vi "GUI_BELLA_PlL2PresCtl.vi"() -> ()   [LabVIEW 2013]
uses:
  Shared/GUI_Template/GUI_master/tcp_new_data_event.ctl
  Shared/GUI_Template/GUI_master/tcp new data cluster.ctl
panel:
  out "tcp data event":T1
  in  "Refresh Button":bool
  in  "Select device":string(combo)="PL1-PresCtl"
  in  "PressureSetPoint.device 2::1":dbl=0.001 caption="Pressure Set Point Plasma1 LP" min=0.0 max=20.0 format="%_4f"
  in  "PressureReading.device 2::1":dbl=0.001 caption="Pressure Reading Plasma1 LP" min=-10.0 max=20.0 format="%_4p"
  in  "stop":bool
  in  "PressureSetPoint.device 1::1":dbl=0.001 caption="Pressure Set Point Plasma1 HP" min=0.0 max=20.0 format="%_4f"
  in  "PressureReading.device 1::1":dbl=0.001 caption="Pressure Reading Plasma1 HP" min=-10.0 max=20.0 format="%_4p"
  in  "GUIdevice 1":string="PL2-PresCtl"
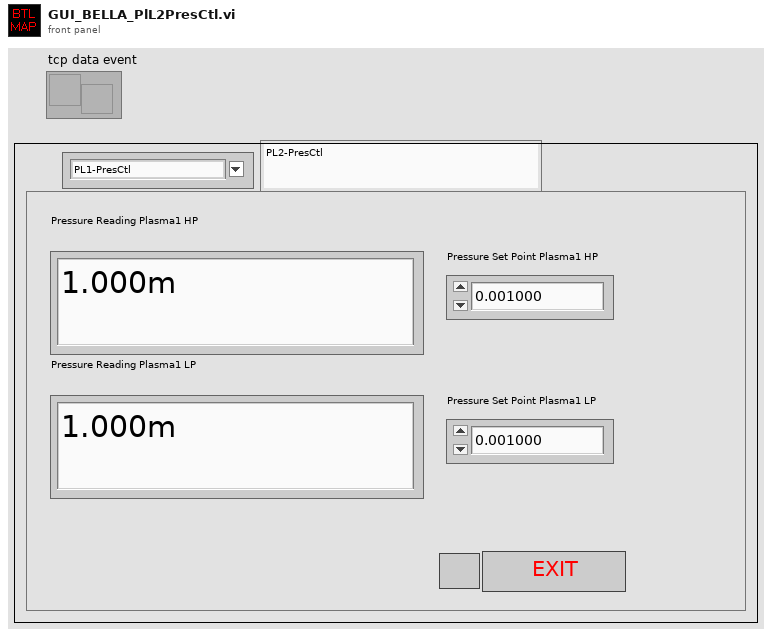
[diagram p1: front panel]
types:
  T1 = typedef "tcp_new_data_event.ctl" = refnum<user-event>
  T2 = enum32{"invalid app kind", "Development System", "Run Time System", "Student Edition", "Embedded LabVIEW", "Evaluation", "Custom"}
  T3 = typedef "tcp new data cluster.ctl" = cluster{"EventEnum":enum16{"new data", "connection status update"}, "Device name":string}
  T4 = enum32{"Invalid", "Standard", "Closed", "Hidden", "Minimized", "Maximized"}
  T5 = cluster{"Core":cluster{"Current VI Reference":refnum<vi>, "Close Panel on Exit?":bool}, "Your Boolean data":bool, "Your string data":string, "SuperGUI":cluster{"STOP queue":refnum<queue>, "SuperGUI ref":refnum<vi>}}
  T6 = cluster{"STOP queue":refnum<queue>, "SuperGUI ref":refnum<vi>}
  T7 = cluster{"Current VI Reference":refnum<vi>, "Close Panel on Exit?":bool}
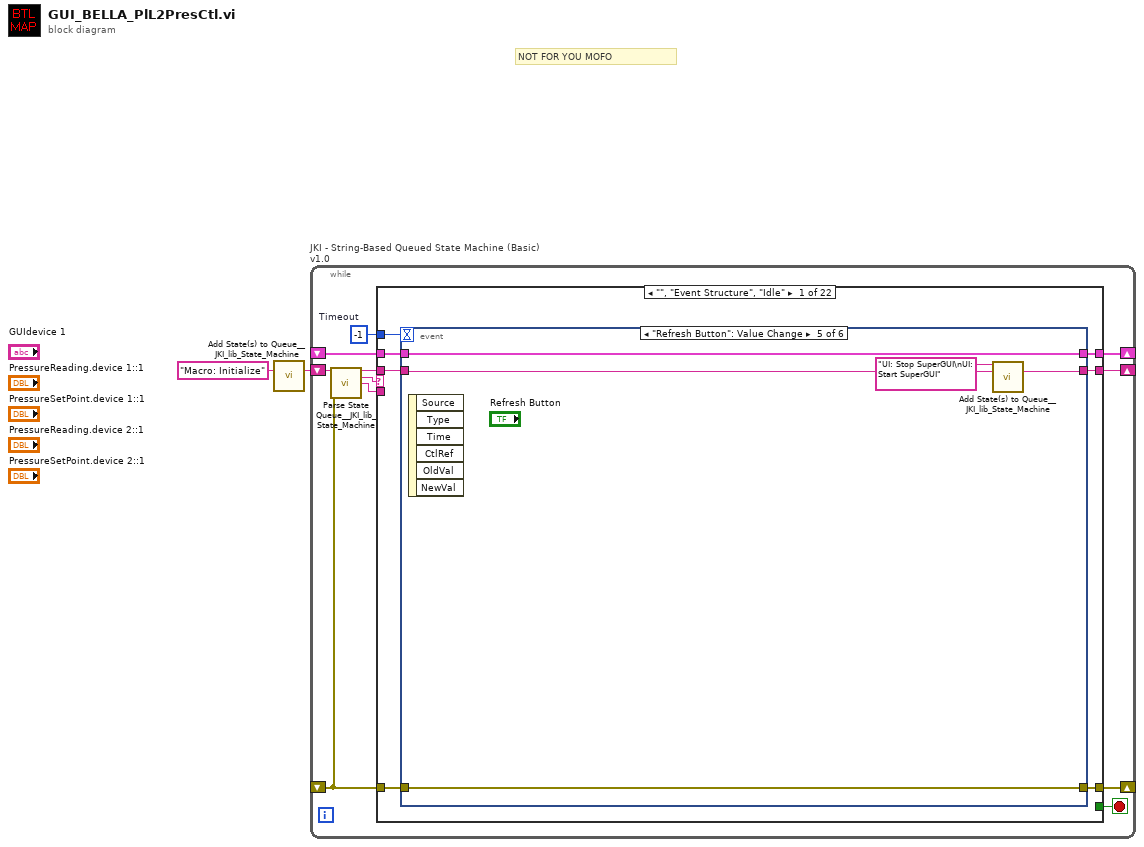
[diagram p0: block diagram]
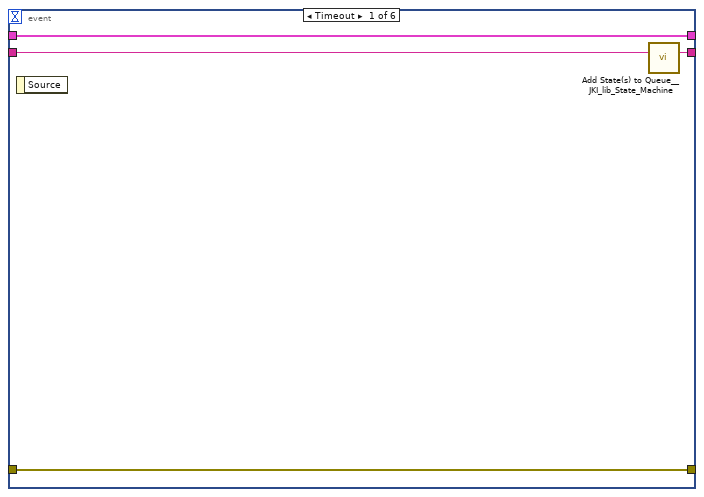
[diagram p2: hidden frame]
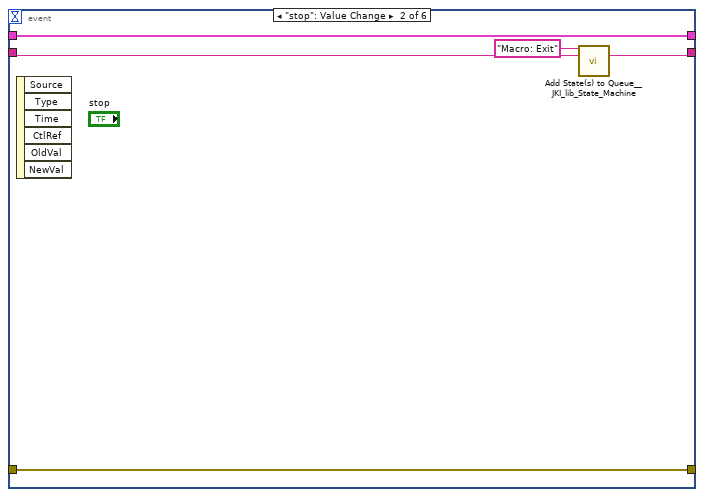
[diagram p3: hidden frame]
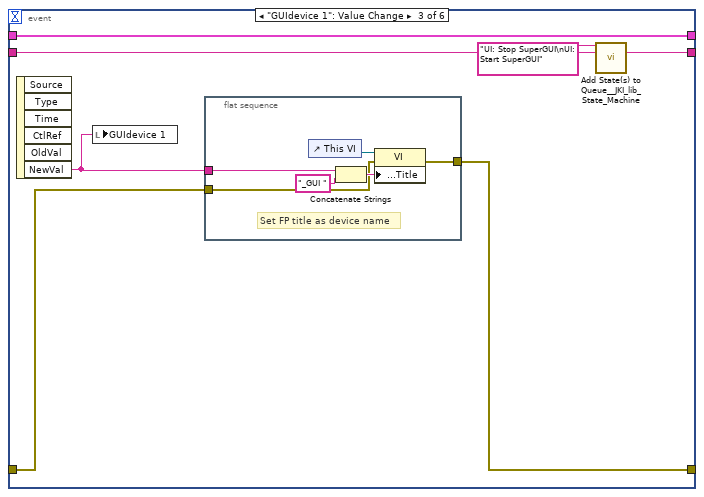
[diagram p4: hidden frame]
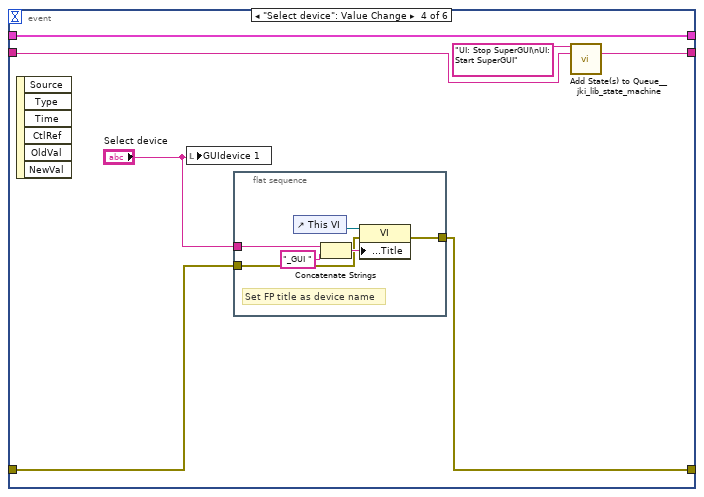
[diagram p5: hidden frame]
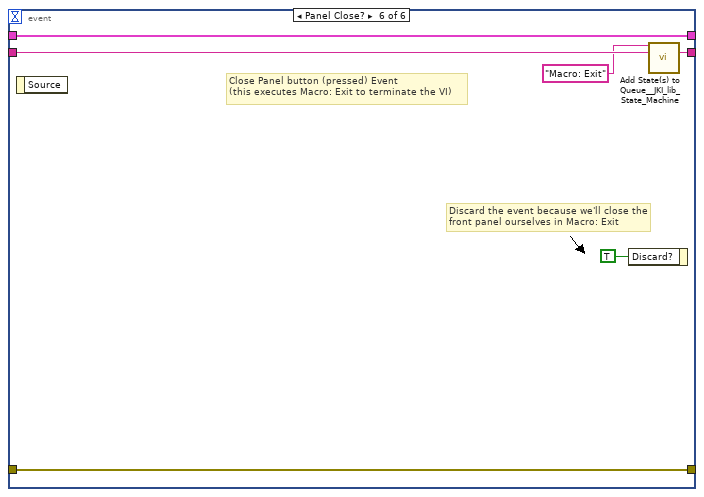
[diagram p6: hidden frame]
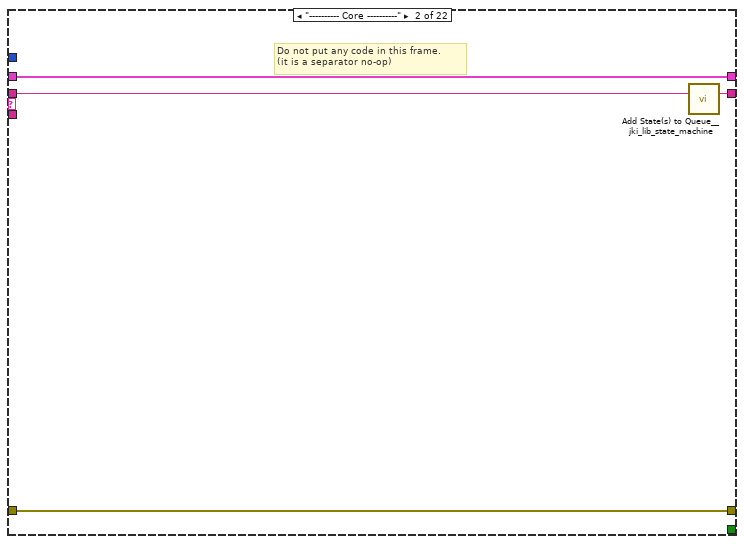
[diagram p7: hidden frame]
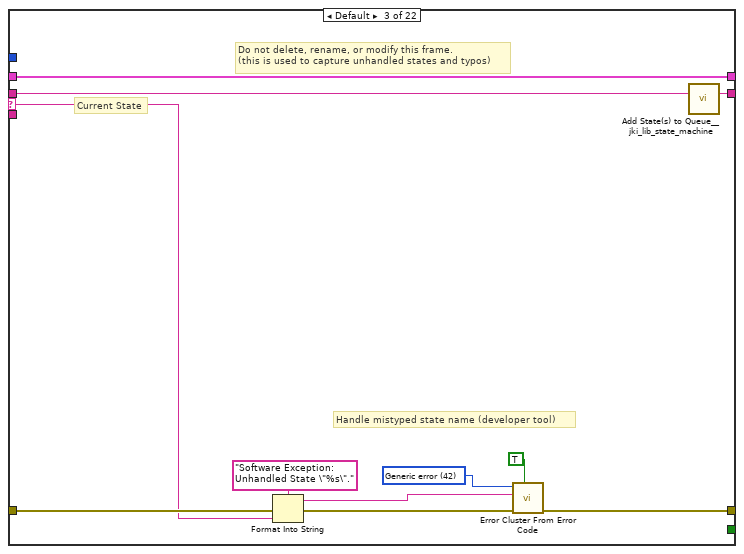
[diagram p8: hidden frame]
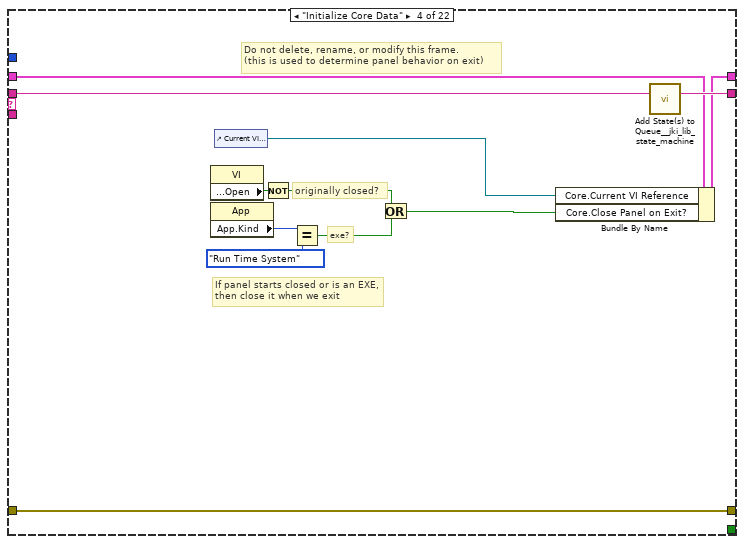
[diagram p9: hidden frame]
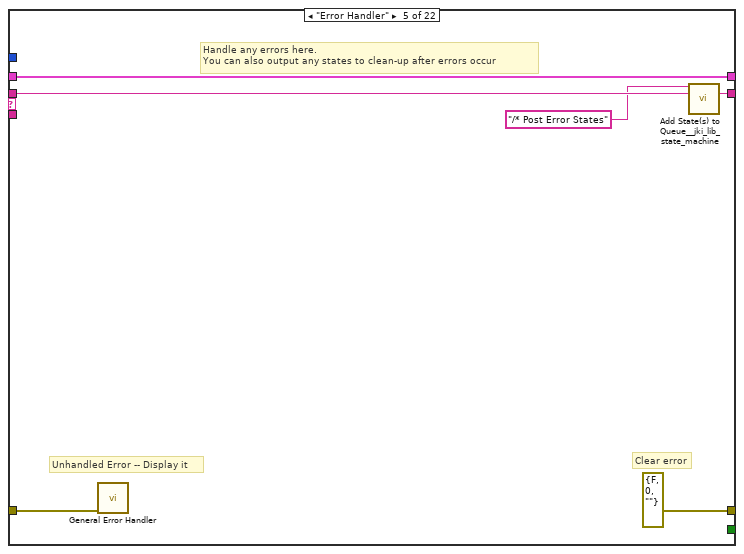
[diagram p10: hidden frame]
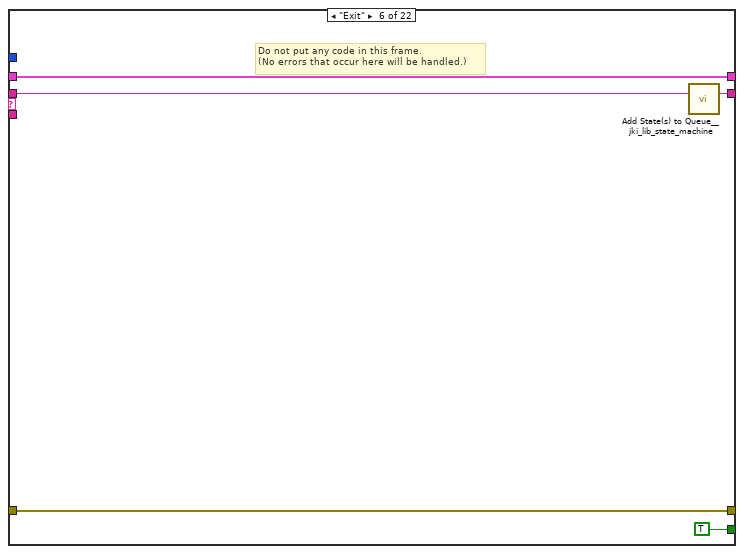
[diagram p11: hidden frame]
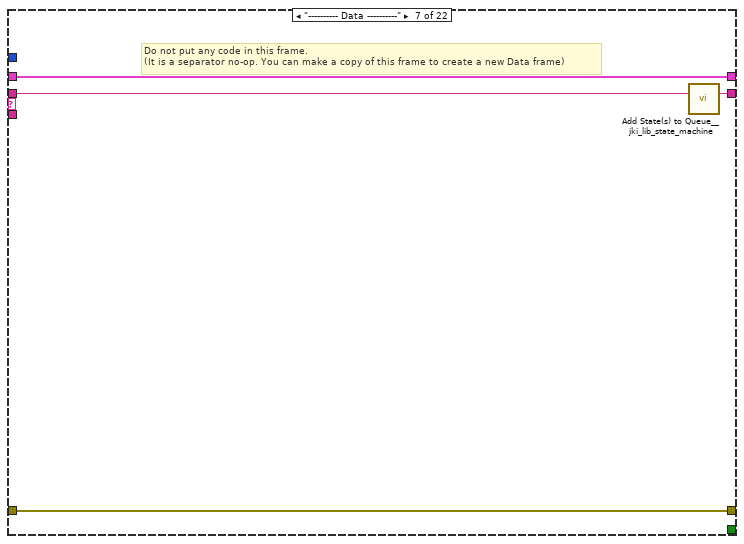
[diagram p12: hidden frame]
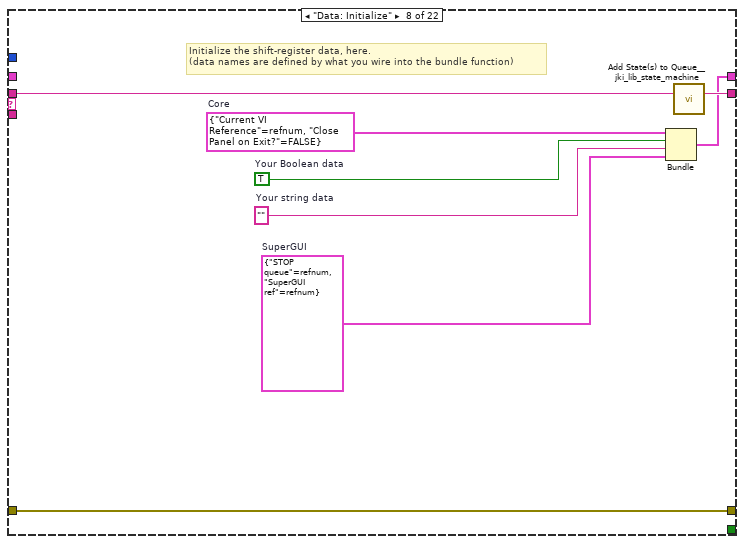
[diagram p13: hidden frame]
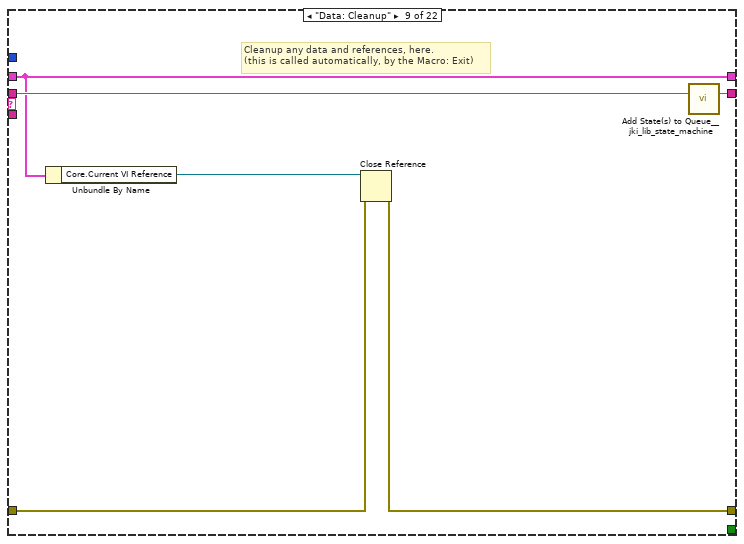
[diagram p14: hidden frame]
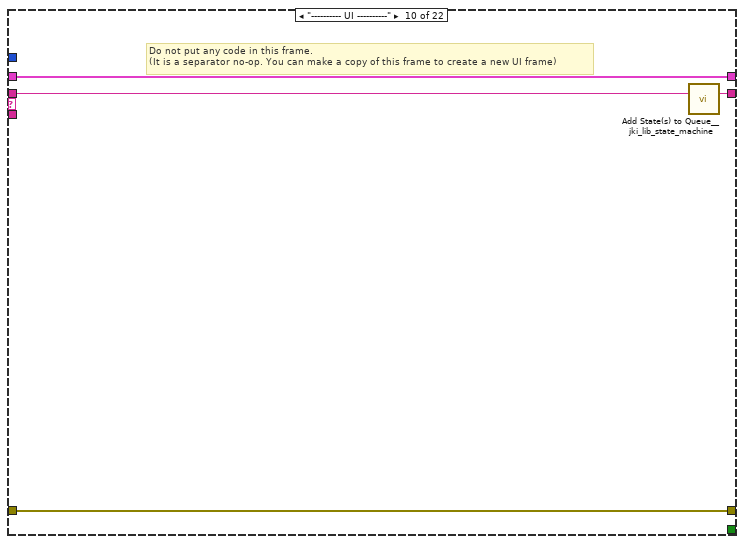
[diagram p15: hidden frame]
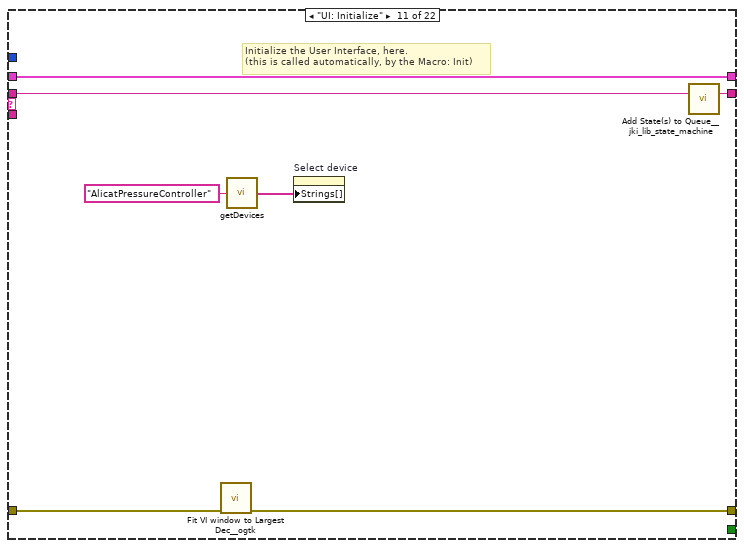
[diagram p16: hidden frame]
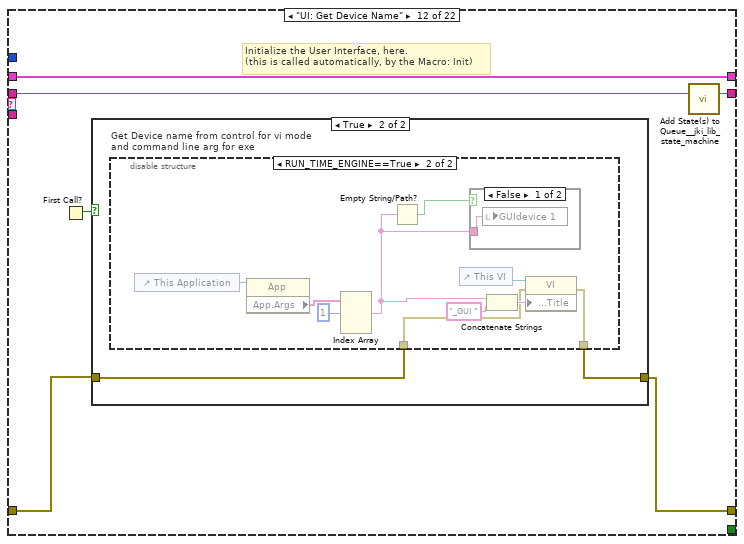
[diagram p17: hidden frame]
diagram:
  # "NOT FOR YOU MOFO"
  n1 = call <vilib>:"Add State(s) to Queue__JKI_lib_State_Machine.vi"("State(s) in (\"\")"="Macro: Initialize") -> ("States Out"=w2:string)  [unwired: 14 in]
  n2 = while "JKI - String-Based Queued State Machine (Basic) v1.0" {
    shift-right: [w6] -> _
    shift-left: _ -> [w5]
    shift-right: [w9] -> _
    shift-left: _ -> [w3]
    shift-right: [w8] -> _
    shift-left: w2 -> [w10]
    stop <- w7 stop-if-true
    w4 = -1  # Timeout
    n3 = call <vilib>:"Parse State Queue__JKI_lib_State_Machine.vi"("State Queue"=w10, "Error In (no error)"=w3) -> ("Remaining States"=w12:string, "Current State"=w13:string, "Arguments"=w11:string)  [unwired: 11 in]
    n4 = case shown="\"\", \"Event Structure\", \"Idle\"" w13 {
      selector: w13 -> [_ _ w71 _ _ _ _ _ _ _ _ _ _ _ _ _ _ _ _ _ _ _]
      tunnel: w12 -> [w20 w70 w75 w93 w99 w104 w108 w116 w122 w126 w133 w139 w174 w182 w188 w199 w225 w230 w240 w244 w248 w252]
      tunnel: w11 -> [_ _ _ _ _ _ _ _ _ _ _ _ _ _ w183 w193 _ _ _ _ _ _]
      tunnel: w5 -> [w18 w67 w73 w84 w96 w102 w105 _ w117 w123 w131 w137 w165 w177 w186 w195 w222 w227 w237 w241 w245 w249]
      tunnel: [w17 w68 w77 w90 errorcluster {"status"=FALSE, "code"=0, "source"=""} ("error out") w101 w106 w113 w118 w124 w127 w134 w158 w175 w184 w196 w223 w228 w238 w242 w246 w250] -> w9
      tunnel: w3 -> [w16 w68 w76 w90 w95 w101 w106 w113 w119 w124 w130 w135 w159 w176 w185 w197 w223 w228 w238 w242 w246 w250]
      tunnel: [w19 w69 w74 w92 w98 w103 w107 w115 w121 w125 w132 w138 w173 w181 w187 w198 w224 w229 w239 w243 w247 w251] -> w8
      tunnel: [_ _ _ _ _ TRUE _ _ _ _ _ _ _ _ _ _ _ _ _ _ _ _] -> w7
      tunnel: [w15 w67 w73 w91 w96 w102 w105 w114 w117 w123 w131 w137 w164 w177 w186 w195 w222 w227 w237 w241 w245 w249] -> w6
      tunnel: w4 -> [w14 _ _ _ _ _ _ _ _ _ _ _ _ _ _ _ _ _ _ _ _ _]
      frame "", "Event Structure", "Idle" {
        n5 = event shown="[4] \"Refresh Button\": Value Change" {
          selector: _ -> [_ _ _ _ _ _]
          dyn-events: _ -> [_ _ _ _ _ _]
          timeout: w14 -> [_ _ _ _ _ _]
          tunnel: w20 -> [w24 w27 w33 w44 w58 w66]
          tunnel: [w23 w26 w32 w43 w57 w65] -> w19
          tunnel: w18 -> [w21 w29 w36 w49 w60 w63]
          tunnel: [w22 w28 w34 w46 w59 w64] -> w17
          tunnel: w16 -> [w22 w28 w35 w47 w59 w64]
          tunnel: [w21 w29 w36 w49 w60 w63] -> w15
          event Timeout {
            n6 = event-data() -> ()  [unwired: 1 in, 1 out]
            n7 = call <vilib>:"Add State(s) to Queue__JKI_lib_State_Machine.vi"("State(s) in (\"\")"=w24) -> ("States Out"=w23:string)  [unwired: 14 in]
          }
          event "stop": Value Change {
            n8 = event-data() -> ()  [unwired: 1 in, 6 out]
            n9 = call <vilib>:"Add State(s) to Queue__JKI_lib_State_Machine.vi"("State(s) in Front (\"\")"="Macro: Exit", "State(s) in (\"\")"=w27) -> ("States Out"=w26:string)  [unwired: 13 in]
          }
          event "GUIdevice 1": Value Change {
            n10 = event-data() -> ("NewVal"=w30:string)  [unwired: 1 in, 5 out]
            n11 = local write "GUIdevice 1"(w30) -> ()
            n12 = flat-sequence {
              tunnel: [w39] -> w34
              tunnel: w35 -> [w38]
              tunnel: w30 -> [w37]
              frame #0 {
                # "Set FP title as device name"
                n13 = control-ref of="This VI"() -> (w42:refnum<vi>)
                n14 = Concatenate Strings(w37, "_GUI ") -> (w41:string)
                n15 = property class="VI"(reference=w42, error in=w38, "Front Panel.Title"=w41) -> (error out=w39:errorcluster)  [unwired: 1 out]
              }
            }
            n16 = call <vilib>:"Add State(s) to Queue__JKI_lib_State_Machine.vi"("State(s) in Front (\"\")"="UI: Stop SuperGUI\nUI: Start SuperGUI", "State(s) in (\"\")"=w33) -> ("States Out"=w32:string)  [unwired: 13 in]
          }
          event "Select device": Value Change {
            n17 = event-data() -> ()  [unwired: 1 in, 6 out]
            n18 = local write "GUIdevice 1"("Select device") -> ()
            n19 = flat-sequence {
              tunnel: [w52] -> w46
              tunnel: w47 -> [w51]
              tunnel: "Select device" -> [w50]
              frame #0 {
                # "Set FP title as device name"
                n20 = control-ref of="This VI"() -> (w55:refnum<vi>)
                n21 = Concatenate Strings(w50, "_GUI ") -> (w54:string)
                n22 = property class="VI"(reference=w55, error in=w51, "Front Panel.Title"=w54) -> (error out=w52:errorcluster)  [unwired: 1 out]
              }
            }
            n23 = call <vilib>:"Add State(s) to Queue__jki_lib_state_machine.vi"("State(s) in Front (\"\")"="UI: Stop SuperGUI\nUI: Start SuperGUI", "State(s) in (\"\")"=w44) -> ("States Out"=w43:string)  [unwired: 13 in]
          }
          event "Refresh Button": Value Change {
            n24 = event-data() -> ()  [unwired: 1 in, 6 out]
            n25 = call <vilib>:"Add State(s) to Queue__JKI_lib_State_Machine.vi"("State(s) in Front (\"\")"="UI: Stop SuperGUI\nUI: Start SuperGUI", "State(s) in (\"\")"=w58) -> ("States Out"=w57:string)  [unwired: 13 in]
          }
          event Panel Close? {
            # "Discard the event because we'll close the front panel ourselves in Macro: Exit"
            # "Close Panel button (pressed) Event\n(this executes Macro: Exit to terminate the VI)"
            n26 = event-data() -> ()  [unwired: 1 in, 1 out]
            n27 = event-data("Discard?"=TRUE) -> ()  [unwired: 1 in, 1 out]
            n28 = call <vilib>:"Add State(s) to Queue__JKI_lib_State_Machine.vi"("State(s) in Front (\"\")"="Macro: Exit", "State(s) in (\"\")"=w66) -> ("States Out"=w65:string)  [unwired: 13 in]
          }
        }
      }
      frame "---------- Core ----------" {
        # "Do not put any code in this frame.\n(it is a separator no-op)"
        n29 = call <vilib>:"Add State(s) to Queue__jki_lib_state_machine.vi"("State(s) in (\"\")"=w70) -> ("States Out"=w69:string)  [unwired: 14 in]
      }
      frame Default {
        w80 = 42 items=["No error", "Argument error", "Memory is full", "Out of zone", "End of file", "File already open", "Generic file I/O error", "File not found", "File permission error", "Disk is full", "Duplicate path", "Too many files open", "System feature not enabled", "Resource file not found", "Cannot add resource", "Resource not found", "Image not found", "Image memory error", "Pen does not exist", "Config type invalid", "Config token not found", "Config parse error", "Config memory error", "Bad external code format", "Bad external code offset", "External code not present", "Null window", "Destroy window error", "Null menu", "Print aborted", "Bad print record", "Print driver error", "Windows error during printing", "Memory error during printing", "Print dialog error", "Generic print error", "Invalid device refnum", "Device not found", "Device parameter error", "Device unit error", "Cannot open device", "Device call aborted", "Generic error", "Cancelled by user", "Object ID too low", "Object ID too high", "Object not in heap", "Unknown heap", "Unknown object (invalid DefProc)", "Unknown object (DefProc not in table)", "Message out of range", "Invalid (null) method", "Unknown message", "Manager call not supported", "Bad address", "Network operation in progress", "Network operation timed out", "Connection is busy", "Network attribute not supported", "Network error", "Address in use", "System out of memory", "Connection aborted", "Connection refused", "Not connected", "Already connected", "Connection closed", "Initialization error (interapplication manager)", "Bad occurrence", "Wait on unbound occurrence handler", "Occurrence queue overflow", "Datalog type conflict", "Unused", "Unrecognized type (interapplication manager)", "Memory corrupt", "Failed to make temporary DLL", "Old CIN version", "Drag socket not found", "Failed to load drop-object", "Failed to register OLE object", "Failed to release OLE object", "Format specifier type mismatch", "Unknown format specifier", "Too few format specifiers", "Too many format specifiers", "Scan failed", "Newer CIN version", "Error converting to variant", "Runtime menu error", "Password tampered", "Variant attribute not found", "Incompatible variant data type", "Event data is not available", "Event Store is not present", "Occurrence is not found", "Event Queue is not created", "Event info is not available", "Refnum passed is NULL", "Error retrieving Class GUID", "Error retrieving CoClass GUID", "Error retrieving TypeLib GUID.", "Bad built application magic bytes.", "Specific driver is different from the specific driver associated with the Logical Name.", "There is no session opened to the class driver.", "Max Error", "MAX - Error with config objects", "MAX - Error loading configuration", "MAX - Group not supported"]
        # "Current State"
        # "Do not delete, rename, or modify this frame.\n(this is used to capture unhandled states and typos)"
        # "Handle mistyped state name (developer tool)"
        n30 = Format Into String(format string="Software Exception: Unhandled State \"%s\"." ("message"), error in=w76, w71) -> (resulting string=w79:string, error out=w78:errorcluster)  [unwired: 1 in]
        n31 = call <vilib>:"Error Cluster From Error Code.vi"("show call chain? (False)"=TRUE, "error in (no error)"=w78, "error message (\"\")"=w79, "error code (0)"=w80) -> ("error out"=w77:errorcluster)  [unwired: 5 in]
        n32 = call <vilib>:"Add State(s) to Queue__jki_lib_state_machine.vi"("State(s) in (\"\")"=w75) -> ("States Out"=w74:string)  [unwired: 14 in]
      }
      frame "Initialize Core Data" {
        # "Do not delete, rename, or modify this frame.\n(this is used to determine panel behavior on exit)"
        # "originally closed?"
        # "exe?"
        # "If panel starts closed or is an EXE, then close it when we exit"
        n33 = property class="VI"() -> ("Front Panel.Open"=w89:bool)  [unwired: 2 in, 2 out]
        n34 = property class="App"() -> ("App.Kind"=w88:T2)  [unwired: 2 in, 2 out]
        n35 = control-ref of="Current VI Reference"() -> (w82:refnum<vi>)
        n36 = Not(x=w89) -> (.not. x?=w86:bool)
        n37 = Equal?(x=w88, y=T2."Run Time System" ("Application:Kind")) -> (x = y?=w85:bool)
        n38 = Or(x=w86, y=w85) -> (x .or. y?=w83:bool)
        n39 = Bundle By Name(cluster=w84, "Core.Current VI Reference"=w82, "Core.Close Panel on Exit?"=w83) -> (w91:T5)
        n40 = call <vilib>:"Add State(s) to Queue__jki_lib_state_machine.vi"("State(s) in (\"\")"=w93) -> ("States Out"=w92:string)  [unwired: 14 in]
      }
      frame "Error Handler" {
        # "Unhandled Error -- Display it"
        # "Handle any errors here.\nYou can also output any states to clean-up after errors occur"
        # "Clear error"
        n41 = call <vilib>:"General Error Handler.vi"("error in (no error)"=w95) -> ()  [unwired: 10 in, 5 out]
        n42 = call <vilib>:"Add State(s) to Queue__jki_lib_state_machine.vi"("State(s) in Front (\"\")"="/* Post Error States", "State(s) in (\"\")"=w99) -> ("States Out"=w98:string)  [unwired: 13 in]
      }
      frame "Exit" {
        # "Do not put any code in this frame.\n(No errors that occur here will be handled.)"
        n43 = call <vilib>:"Add State(s) to Queue__jki_lib_state_machine.vi"("State(s) in (\"\")"=w104) -> ("States Out"=w103:string)  [unwired: 14 in]
      }
      frame "---------- Data ----------" {
        # "Do not put any code in this frame.\n(It is a separator no-op. You can make a copy of this frame to create a new Data frame)"
        n44 = call <vilib>:"Add State(s) to Queue__jki_lib_state_machine.vi"("State(s) in (\"\")"=w108) -> ("States Out"=w107:string)  [unwired: 14 in]
      }
      frame "Data: Initialize" {
        w109 = T6 {"STOP queue"=refnum, "SuperGUI ref"=refnum}  # SuperGUI
        w110 = T7 {"Current VI Reference"=refnum, "Close Panel on Exit?"=FALSE}  # Core
        w112 = TRUE  # Your Boolean data
        w111 = ""  # Your string data
        # "Initialize the shift-register data, here.\n(data names are defined by what you wire into the bundle function)"
        n45 = Bundle("Core"=w110, "Your Boolean data"=w112, "Your string data"=w111, "SuperGUI"=w109) -> (w114:T5)  [unwired: 1 in]
        n46 = call <vilib>:"Add State(s) to Queue__jki_lib_state_machine.vi"("State(s) in (\"\")"=w116) -> ("States Out"=w115:string)  [unwired: 14 in]
      }
      frame "Data: Cleanup" {
        # "Cleanup any data and references, here.\n(this is called automatically, by the Macro: Exit)"
        n47 = Unbundle By Name(w117) -> ("Core.Current VI Reference"=w120:refnum<vi>)
        n48 = Close Reference(reference=w120, error in (no error)=w119) -> (error out=w118:errorcluster)
        n49 = call <vilib>:"Add State(s) to Queue__jki_lib_state_machine.vi"("State(s) in (\"\")"=w122) -> ("States Out"=w121:string)  [unwired: 14 in]
      }
      frame "---------- UI ----------" {
        # "Do not put any code in this frame.\n(It is a separator no-op. You can make a copy of this frame to create a new UI frame)"
        n50 = call <vilib>:"Add State(s) to Queue__jki_lib_state_machine.vi"("State(s) in (\"\")"=w126) -> ("States Out"=w125:string)  [unwired: 14 in]
      }
      frame "UI: Initialize" {
        # "Initialize the User Interface, here.\n(this is called automatically, by the Macro: Init)"
        n51 = call <userlib>:"Fit VI window to Largest Dec__ogtk.vi"("error in (no error)"=w130) -> ("error out"=w127:errorcluster)  [unwired: 5 in, 1 out]
        n52 = call "getDevices.vi"("Device Class"="AlicatPressureController") -> ("All Devices"=w128:string[])
        n53 = property on="Select device" class="CmbBox"("Strings[]"=w128) -> ()  [unwired: 2 in, 2 out]
        n54 = call <vilib>:"Add State(s) to Queue__jki_lib_state_machine.vi"("State(s) in (\"\")"=w133) -> ("States Out"=w132:string)  [unwired: 14 in]
      }
      frame "UI: Get Device Name" {
        # "Initialize the User Interface, here.\n(this is called automatically, by the Macro: Init)"
        n55 = First Call?() -> (First Call?: T/F=w136:bool)
        n56 = case shown="True" w136 {
          tunnel: w135 -> [w140 w142]
          tunnel: [w140 w141] -> w134
          frame False {
          }
          frame True {
            n57 = disable-structure "Get Device name from control for vi mode\nand command line arg for exe" shown="RUN_TIME_ENGINE==True" {
              disable-tunnel: w142 -> [w143 w145]
              disable-tunnel: [w143 w144] -> w141
              frame condition #0 (active) {
              }
              frame condition #1 {
                n58 = control-ref of="This Application"() -> (w153:refnum<vi>)
                n59 = property class="App"(reference=w153) -> ("App.Args"=w152:string[])  [unwired: 1 in, 2 out]
                n60 = Index Array(array=w152, index #1=1 ("index")) -> (element #1=w146:string)  [unwired: 2 in, 2 out]
                n61 = Empty String/Path?(string/path=w146) -> (empty?=w150:bool)
                n62 = control-ref of="This VI"() -> (w149:refnum<vi>)
                n63 = case shown="False" w150 {
                  tunnel: w146 -> [w154 _]
                  frame False {
                    n64 = local write "GUIdevice 1"(w154) -> ()
                  }
                  frame True {
                  }
                }
                n65 = Concatenate Strings(w146, "_GUI ") -> (w148:string)
                n66 = property class="VI"(reference=w149, error in=w145, "Front Panel.Title"=w148) -> (error out=w144:errorcluster)  [unwired: 1 out]
              }
            }
          }
        }
        n67 = call <vilib>:"Add State(s) to Queue__jki_lib_state_machine.vi"("State(s) in (\"\")"=w139) -> ("States Out"=w138:string)  [unwired: 14 in]
      }
      frame "UI: Start SuperGUI" {
        # "create stop queue for supergui and its clones"
        # "x100 abort will be dependent on caller VI\nx80 abort will be independent of caller vi, this will abort vi when labview is closed."
        # "Start SuperGUI asynchronous way"
        n68 = vi-ref "GUI_Master_subvi_reentrant_queues.vi"() -> (w157:refnum<vi>)
        n69 = property class="VI"(reference=w157) -> ("Path"=w156:path)  [unwired: 1 in, 2 out]
        n70 = Create User Event(user event datatype=T3 {"EventEnum"=enum."new data", "Device name"="Device name"} ("New Event"), error in=w159) -> (user event=w160:refnum<user-event>, error out=w166:errorcluster)
        "tcp data event" <- w160
        n71 = control-ref of="This Application"() -> (w163:refnum<vi>)
        n72 = control-ref of="This VI"() -> (w162:refnum<vi>)
        n73 = Open VI Reference(type specifier VI Refnum (for type only)=refnum<vi> refnum, vi path=w156, options=256) -> (vi reference=w172:refnum<vi>, error out=w171:errorcluster)  [unwired: 3 in]
        n74 = register-events(w160) -> ()  [unwired: 2 in, 2 out]
        n75 = call "supergui create stop queue.vi"() -> ("STOP Queue out"=w168:refnum<queue>)  [unwired: 11 in]
        n76 = Current VI's Menubar() -> (w161:refnum<k9>)
        n77 = call-by-ref "Start Asynchronous Call"(reference=w172, error in=w171, "STOP Queue in"=w168, "This Application"=w163, 8:"error in (no error)"=w166, "tcp data event"=w160, "Caller menu reference"=w161, "Caller VI ref"=w162) -> (reference out=w155:refnum<vi>, error out=w158:errorcluster)  [unwired: 5 in, 1 out]
        n78 = Bundle By Name(cluster=w165, "SuperGUI.SuperGUI ref"=w155, "SuperGUI.STOP queue"=w168) -> (w164:T5)
        n79 = call <vilib>:"Add State(s) to Queue__jki_lib_state_machine.vi"("State(s) in (\"\")"=w174) -> ("States Out"=w173:string)  [unwired: 14 in]
      }
      frame "UI: Stop SuperGUI" {
        # "Stop Supergui Clone and wait until it exit properly"
        n80 = Unbundle By Name(w177) -> ("SuperGUI.SuperGUI ref"=w179:refnum<vi>, "SuperGUI.STOP queue"=w178:refnum<queue>)
        n81 = Release Queue(queue=w178, error in (no error)=w176) -> (error out=w180:errorcluster)  [unwired: 1 in, 2 out]
        n82 = call-by-ref "Wait On Asynchronous Call"(reference=w179, error in=w180) -> ("error out"=w175:errorcluster)  [unwired: 11 in, 2 out]
        n83 = call <vilib>:"Add State(s) to Queue__jki_lib_state_machine.vi"("State(s) in (\"\")"=w182) -> ("States Out"=w181:string)  [unwired: 14 in]
      }
      frame "UI: Cursor Set" {
        # "Argument"
        # "Set and Unset Cursor Busy.\n(Usage: \"UI: Cursor Set >> Busy|Idle\")"
        n84 = case shown="\"Idle\", Default" w183 {
          tunnel: w185 -> [w190 w192]
          tunnel: [w189 w191] -> w184
          frame "Idle", Default {
            n85 = call <vilib>:"Unset Busy.vi"("error in (no error)"=w190) -> ("error out"=w189:errorcluster)  [unwired: 10 in]
          }
          frame "Busy" {
            n86 = call <vilib>:"Set Busy.vi"("error in (no error)"=w192) -> ("error out"=w191:errorcluster)  [unwired: 9 in, 1 out]
          }
        }
        n87 = call <vilib>:"Add State(s) to Queue__jki_lib_state_machine.vi"("State(s) in (\"\")"=w188) -> ("States Out"=w187:string)  [unwired: 14 in]
      }
      frame "UI: Front Panel State" {
        # "Argument"
        # "Set Front Panel Open or Closed\n(Usage: \"UI: Front Panel State >> Open|Close\")"
        n88 = Unbundle By Name(w195) -> ("Core.Current VI Reference"=w194:refnum<vi>)
        n89 = case shown="\"Open\", Default" w193 {
          tunnel: w197 -> [w203 w216]
          tunnel: [w205 w217] -> w196
          tunnel: w194 -> [w204 w214]
          frame "Open", Default {
            n90 = property class="VI"(reference=w204, error in=w203) -> (reference out=w201:refnum<vi>, error out=w202:errorcluster, "Front Panel.Open"=w200:bool)
            n91 = case shown="False" w200 {
              tunnel: [w208 w211] -> w205
              tunnel: w202 -> [w207 w211]
              tunnel: w201 -> [w206 _]
              frame False {
                n92 = invoke class="VI" method="FP.Open"(reference=w206, error in=w207, "Activate"=TRUE, "State"=T4."Standard") -> (error out=w208:errorcluster)  [unwired: 1 in, 4 out]
              }
              frame True {
              }
            }
          }
          frame "Close" {
            n93 = property class="VI"(reference=w214, error in=w216) -> (reference out=w213:refnum<vi>, error out=w215:errorcluster, "Front Panel.Open"=w212:bool)
            n94 = case shown="True" w212 {
              tunnel: [w218 w221] -> w217
              tunnel: w215 -> [w218 w220]
              tunnel: w213 -> [_ w219]
              frame False {
              }
              frame True {
                n95 = invoke class="VI" method="FP.Close"(reference=w219, error in=w220) -> (error out=w221:errorcluster)  [unwired: 1 in, 2 out]
              }
            }
          }
        }
        n96 = call <vilib>:"Add State(s) to Queue__jki_lib_state_machine.vi"("State(s) in (\"\")"=w199) -> ("States Out"=w198:string)  [unwired: 14 in]
      }
      frame "---------- Macro ----------" {
        # "Do not put any code in this frame.\n(It is a separator no-op. You can make a copy of this frame to create a new Macro frame)"
        n97 = call <vilib>:"Add State(s) to Queue__jki_lib_state_machine.vi"("State(s) in (\"\")"=w225) -> ("States Out"=w224:string)  [unwired: 14 in]
      }
      frame "Macro: Initialize" {
        # "Initialization Macro\n(This is called once, when the VI starts)"
        n98 = call <vilib>:"Add State(s) to Queue__jki_lib_state_machine.vi"("State(s) in Front (\"\")"="Data: Initialize\nInitialize Core Data\nUI: Initialize\nUI: Get Device Name\nUI: Start SuperGUI\nUI: Front Panel State >> Open", "State(s) in (\"\")"=w230) -> ("States Out"=w229:string)  [unwired: 13 in]
      }
      frame "Macro: Exit" {
        # "Exit Macro\n(This is called once, when the VI exits)"
        n99 = Unbundle By Name(w237) -> ("Core.Close Panel on Exit?"=w236:bool)
        n100 = Select(t="UI: Front Panel State >> Close", s=w236, f="") -> (s? t:f=w233:string)
        n101 = call <vilib>:"Add State(s) to Queue__jki_lib_state_machine.vi"("State(s) in (\"\")"=w233, "State(s) at Back (\"\")"="Data: Cleanup\nExit") -> ("States Out"=w231:string)  [unwired: 13 in]
        n102 = call <vilib>:"Add State(s) to Queue__jki_lib_state_machine.vi"("State(s) in Front (\"\")"=w231, "State(s) in (\"\")"=w240) -> ("States Out"=w239:string)  [unwired: 13 in]
      }
      frame "---------- New Category ----------" {
        # "Template Separator\n(You can make a copy of, or modify, this frame)"
        n103 = call <vilib>:"Add State(s) to Queue__jki_lib_state_machine.vi"("State(s) in (\"\")"=w244) -> ("States Out"=w243:string)  [unwired: 14 in]
      }
      frame "New Category: 1" {
        # "Your code here.\n(You can make a copy of, or modify, this frame)"
        n104 = call <vilib>:"Add State(s) to Queue__jki_lib_state_machine.vi"("State(s) in (\"\")"=w248) -> ("States Out"=w247:string)  [unwired: 14 in]
      }
      frame "New Category: 2" {
        # "Your code here.\n(You can make a copy of, or modify, this frame)"
        n105 = call <vilib>:"Add State(s) to Queue__jki_lib_state_machine.vi"("State(s) in (\"\")"=w252) -> ("States Out"=w251:string)  [unwired: 14 in]
      }
    }
  }
